vi "add_system_path.vi"(8 "error in (no error)":errorcluster) -> (0 "error out":errorcluster)   [LabVIEW 2015, in "lv-bin-7zip.lvlib"]
uses:
  lv-bin-7zip.lvlib
  private/_controls/files.ctl
  <userlib>/antonio-alexander/lv-bin/public/api/v1/advanced/add_data_path_system.vi
  <userlib>/antonio-alexander/lv-bin/public/api/v1/v1.lvlib
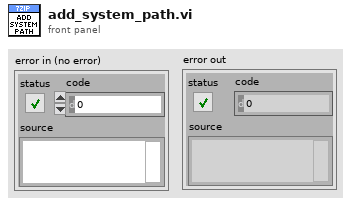
[diagram p1: front panel]
types:
  T1 = typedef "lv-bin-7zip.lvlib/files.ctl" = enum16{"<7z_file>", "7z.dll", "7z.exe", "7z.sfx", "7zCon.sfx", "7zFM. exe", "7zG.exe"}
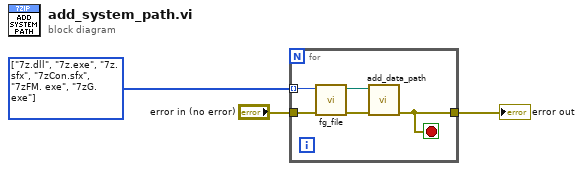
[diagram p0: block diagram]
diagram:
  w3 = T1[] [enum."7z.dll", enum."7z.exe", enum."7z.sfx", enum."7zCon.sfx", enum."7zFM. exe", enum."7zG.exe"] items=["<7z_file>", "7z.dll", "7z.exe", "7z.sfx", "7zCon.sfx", "7zFM. exe", "7zG.exe"]
  n1 = for {
    tunnel: w3 -> [w8] mode=indexing
    tunnel: "error in (no error)" -> [w7]
    tunnel: [w5] -> w1
    stop <- w5 stop-if-true
    n2 = call "fg_file.vi"("error in (no error)"=w7, "files"=w8) -> ("error out"=w6:errorcluster, "file"=w4:path)  [unwired: 8 in]
    n3 = call-poly <userlib>:"add_data_path.vi"("error in (no error)"=w6, "relative_path_file"=w4) -> ("error out"=w5:errorcluster)  [unwired: 9 in]
  }
  "error out" <- w1
